vi "Psychrmoetric Chart by RH.vi"() -> (0 "Psych Chart by RH":dbl[][](array[numeric]))   [LabVIEW 2020]
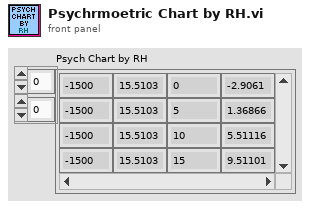
[diagram p1: front panel]
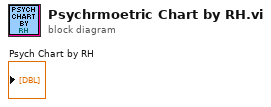
[diagram p0: block diagram]
diagram:
